vi "Chapter2.vi"() -> ()   [LabVIEW 2014]
panel:
  out "Waveform Graph":cluster{i32, dbl, dbl[]}(graph)
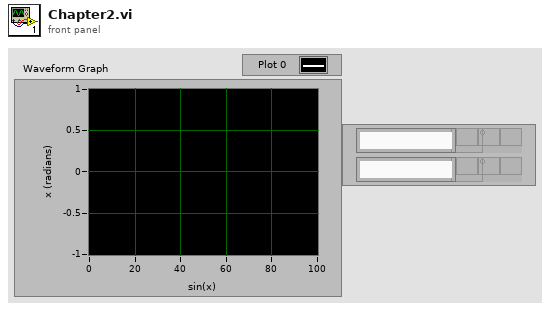
[diagram p1: front panel]
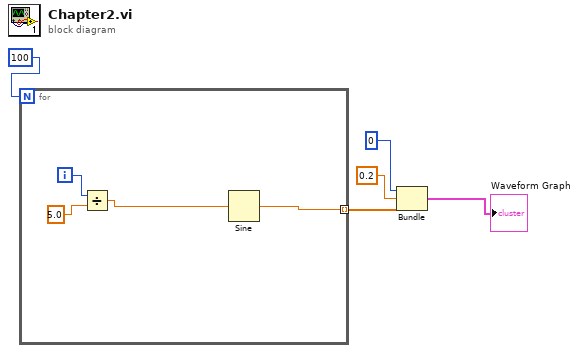
[diagram p0: block diagram]
diagram:
  n1 = for {
    N: 100 ("x/y") -> [_]
    tunnel: [w6] -> w4 mode=indexing
    i -> [w9]
    n2 = Divide(x=w9, y=5.0 ("x/y")) -> (x/y=w8:dbl)
    n3 = Sine(x=w8) -> (sin(x)=w6:dbl)
  }
  n4 = Bundle(0, 0.2, w4) -> (→"Waveform Graph":cluster{i32, dbl, dbl[]})  [unwired: 1 in]
